vi "Create.vi"(8 "error in (no error)":errorcluster, 11 "Core Transfer User Interface in":refnum<class "Core Transfer User Interface.lvclass">) -> (0 "error out":errorcluster, 3 "Core Transfer User Interface out":refnum<class "Core Transfer User Interface.lvclass">)   [LabVIEW 2017, in "DSF Core.lvlib" / "Core Transfer User Interface.lvclass"]
uses:
  Core Transfer User Interface.lvclass
  C:/Git/DSF/Core/Classes/User Interface/User Interface.lvclass
  Configuration/Core/Transfer/Core Transfers Configuration.lvclass
  C:/Git/DSF/Core/Classes/Configuration/Configuration.lvclass
  User Interface.vi
  User Interface.lvclass
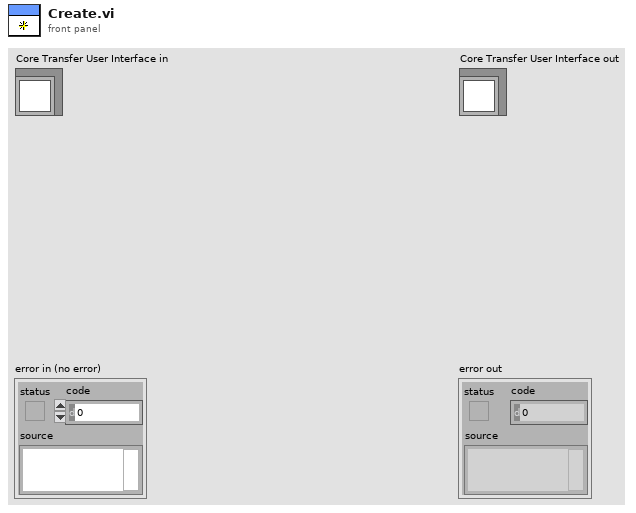
[diagram p1: front panel]
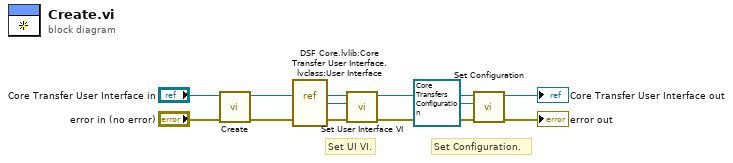
[diagram p0: block diagram]
diagram:
  # "Set Configuration."
  # "Set UI VI."
  n1 = call-parent "Create.vi"("error in (no error)"="error in (no error)", "User Interface in"="Core Transfer User Interface in") -> ("error out"=w10:errorcluster, "User Interface out"=w9:refnum<class "Core Transfer User Interface.lvclass">)  [unwired: 8 in]
  n2 = vi-ref "DSF Core.lvlib:Core Transfer User Interface.lvclass:User Interface.vi"() -> (w5:refnum<vi>)
  n3 = call "Set User Interface VI.vi"("error in (no error)"=w10, "vi"=w5, "User Interface in"=w9) -> ("error out"=w8:errorcluster, "User Interface out"=w7:refnum<class "Core Transfer User Interface.lvclass">)  [unwired: 7 in]
  n4 = call "Set Configuration.vi"("error in (no error)"=w8, "configuration"=refnum<class "Core Transfers Configuration.lvclass"> refnum ("DSF Core.lvlib:Core Transfers Configuration.lvclass"), "User Interface in"=w7) -> ("error out"=→"error out":errorcluster, "User Interface out"=→"Core Transfer User Interface out":refnum<class "Core Transfer User Interface.lvclass">)  [unwired: 7 in]
